vi "CRYGet Graph Data.vi"(11 "pGraph VI":refnum<vi>) -> (0 "Item Symbols":i32[](array[numeric]), 1 "Value Rows":i32[](array[numeric]), 2 "Rows":i32[](array[numeric]), 3 "Type Out":enum16{"Curves", "Values", "Results", "WFM"}(ring), 4 "Result Rows":i32[](array[numeric]))   [LabVIEW 2013]
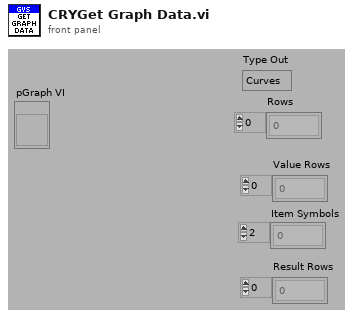
[diagram p1: front panel]
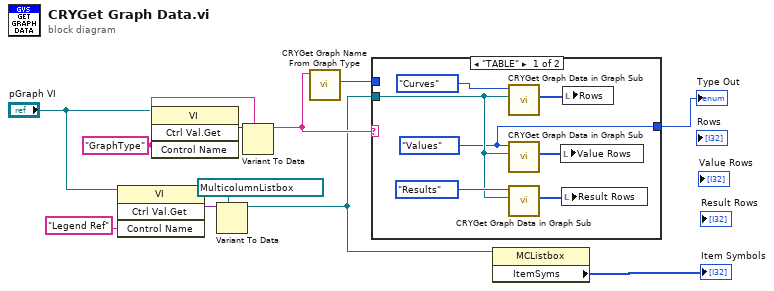
[diagram p0: block diagram]
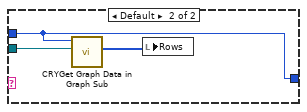
[diagram p2: hidden frame]
diagram:
  w4 = "GraphType" ("Control Name")
  n1 = invoke class="VI" method="Ctrl Val.Get"(reference="pGraph VI", "Control Name"="Legend Ref") -> ("Get Control Value Variant"=w7:variant)  [unwired: 2 in, 3 out]
  n2 = invoke class="VI" method="Ctrl Val.Get"(reference="pGraph VI", "Control Name"=w4) -> ("Get Control Value Variant"=w5:variant)  [unwired: 2 in, 3 out]
  n3 = Variant To Data(type=refnum<vi> refnum ("GMListbox"), Variant=w7) -> (data=w1:refnum<vi>)  [unwired: 1 in, 1 out]
  n4 = Variant To Data(type=w4, Variant=w5) -> (data=w2:string)  [unwired: 1 in, 1 out]
  n5 = call "CRYGet Graph Name From Graph Type.vi"("Graph Type"=w2) -> ("Type"=w11:enum16{"Curves", "Values", "Results", "WFM"})  [unwired: 9 in, 1 out]
  n6 = case shown="\"TABLE\"" w2 {
    tunnel: w1 -> [w16 w21]
    tunnel: w11 -> [_ w19]
    tunnel: [w12 w19] -> w10
    frame "TABLE" {
      w12 = enum16{"Curves", "Values", "Results", "WFM"}."Values" ("Type In")
      n7 = call "CRYGet Graph Data in Graph Sub.vi"("Legend Refnum"=w16, "Type In"=enum16{"Curves", "Values", "Results", "WFM"}."Curves" ("Type")) -> ("Rows"=w15:i32[])  [unwired: 5 in, 4 out]
      n8 = call "CRYGet Graph Data in Graph Sub.vi"("Legend Refnum"=w16, "Type In"=w12) -> ("Rows"=w14:i32[])  [unwired: 5 in, 4 out]
      n9 = call "CRYGet Graph Data in Graph Sub.vi"("Legend Refnum"=w16, "Type In"=enum16{"Curves", "Values", "Results", "WFM"}."Results") -> ("Rows"=w13:i32[])  [unwired: 5 in, 4 out]
      n10 = local write "Value Rows"(w14) -> ()
      n11 = local write "Result Rows"(w13) -> ()
      n12 = local write "Rows"(w15) -> ()
    }
    frame Default {
      n13 = call "CRYGet Graph Data in Graph Sub.vi"("Legend Refnum"=w21, "Type In"=w19) -> ("Rows"=w20:i32[])  [unwired: 5 in, 4 out]
      n14 = local write "Rows"(w20) -> ()
    }
  }
  "Type Out" <- w10
  n15 = property class="MCListbox"(reference=w1) -> ("ItemSyms"=→"Item Symbols":i32[])  [unwired: 1 in, 2 out]
